vi "XML_Get Element Value.vi"(8 "错误输入（无错误）":errorcluster, 11 "引用句柄输入":refnum<k20>) -> (0 "错误输出":errorcluster, 1 "exist?":bool, 2 "value out":string)   [LabVIEW 2016]
uses:
  <resource>/objmgr/DOMUserDefRef.rc
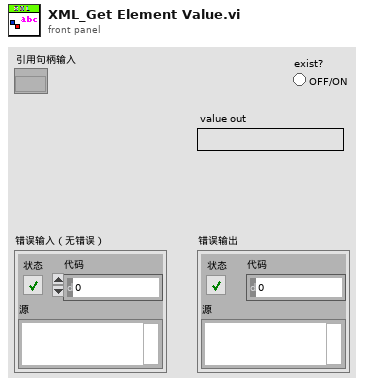
[diagram p1: front panel]
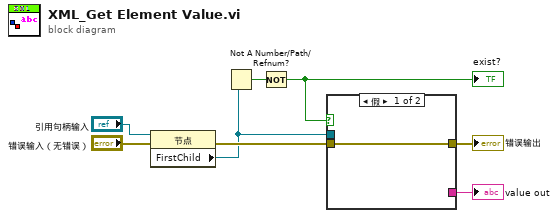
[diagram p0: block diagram]
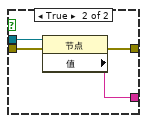
[diagram p2: hidden frame]
diagram:
  n1 = property on="属性节点" class="节点"(reference="引用句柄输入", error in="错误输入（无错误）") -> (error out=w6:errorcluster, "FirstChild"=w5:refnum<k20>)  [unwired: 1 out]
  n2 = Not A Number/Path/Refnum?(number/path/refnum=w5) -> (NaN/Path/Refnum?=w4:bool)
  n3 = Not(x=w4) -> (.not. x?=w3:bool)
  "exist?" <- w3
  n4 = case shown="假" w3 {
    tunnel: [w9 w13] -> w8
    tunnel: [_ w12] -> w7
    tunnel: w6 -> [w9 w11]
    tunnel: w5 -> [_ w10]
    frame False {
    }
    frame True {
      n5 = property on="属性节点" class="节点"(reference=w10, error in=w11) -> (error out=w13:errorcluster, "值"=w12:string)  [unwired: 1 out]
    }
  }
  "错误输出" <- w8
  "value out" <- w7
